vi "wr_xively_one_element.vi"(1 "VALUE":dbl, 2 "Xively_name":string) -> ()   [LabVIEW 2012]
uses:
  <vilib>/httpClient/LabVIEWHTTPClient.lvlib
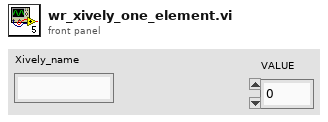
[diagram p1: front panel]
types:
  T1 = typedef "LabVIEWHTTPClient.lvlib/ClientHandle.ctl" = refnum<k1>
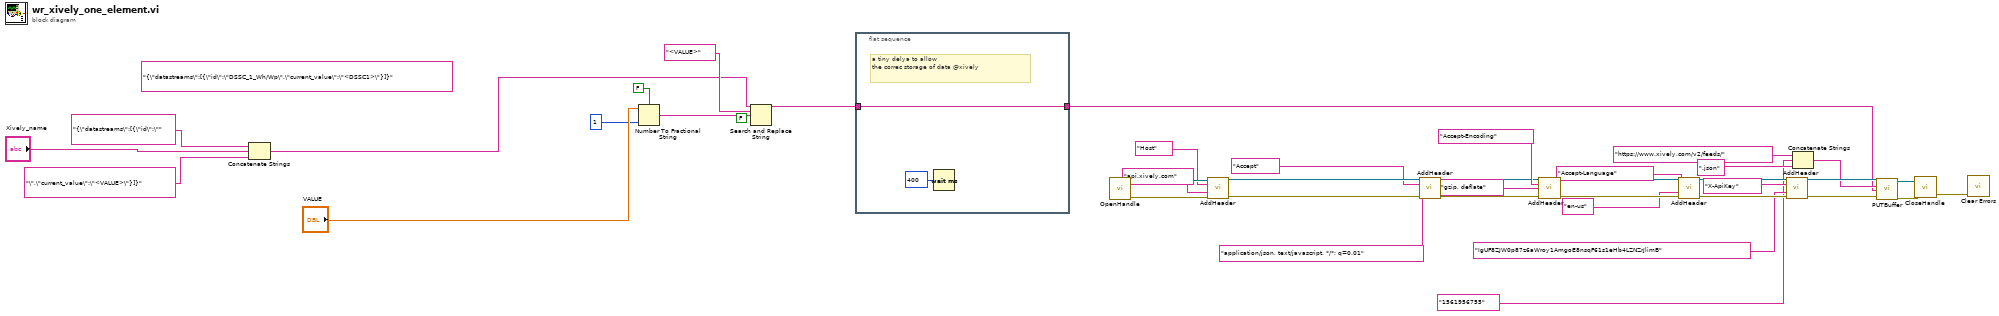
[diagram p0: block diagram]
diagram:
  (unwired) FALSE ("use system decimal point (T)")
  (unwired) "{\"datastreams\":[{\"id\":\"DSSC_1_Wh/Wp\",\"current_value\":\"<DSSC1>\"}]}" ("input string")
  n1 = Concatenate Strings("{\"datastreams\":[{\"id\":\"" ("input string"), "Xively_name", "\",\"current_value\":\"<VALUE>\"}]}" ("input string")) -> (w3:string)
  n2 = Number To Fractional String(use system decimal point (T)=FALSE, number="VALUE", precision (6)=i16 1) -> (F-format string=w18:string)  [unwired: 1 in]
  n3 = Search and Replace String(input string=w3, search string="<VALUE>", replace string=w18) -> (result string=w2:string)  [unwired: 5 in, 3 out]
  n4 = flat-sequence {
    tunnel: w2 -> [w42]
    tunnel: [w42] -> w1
    frame #0 {
      # "a tiny delya to allow\nthe correc storage of data @xively"
      n5 = Wait (ms)(milliseconds to wait=u32 400) -> ()  [unwired: 1 out]
    }
  }
  n6 = call <vilib>:"OpenHandle.vi"() -> ("client handle out"=w36:T1, "error out"=w35:errorcluster)  [unwired: 14 in]
  n7 = call <vilib>:"AddHeader.vi"("client handle"=w36, "header"="Host", "value"="api.xively.com", "error in (no error)"=w35) -> ("client handle out"=w32:T1, "error out"=w31:errorcluster)  [unwired: 10 in]
  n8 = call <vilib>:"AddHeader.vi"("client handle"=w32, "header"="Accept", "value"="application/json, text/javascript, */*; q=0.01", "error in (no error)"=w31) -> ("client handle out"=w27:T1, "error out"=w26:errorcluster)  [unwired: 10 in]
  n9 = call <vilib>:"AddHeader.vi"("client handle"=w27, "header"="Accept-Encoding", "value"="gzip, deflate", "error in (no error)"=w26) -> ("client handle out"=w24:T1, "error out"=w23:errorcluster)  [unwired: 10 in]
  n10 = call <vilib>:"AddHeader.vi"("client handle"=w24, "header"="Accept-Language", "value"="en-us", "error in (no error)"=w23) -> ("client handle out"=w20:T1, "error out"=w19:errorcluster)  [unwired: 10 in]
  n11 = call <vilib>:"AddHeader.vi"("client handle"=w20, "header"="X-ApiKey", "value"="IgUF8ZJW0p87z6aWroy1AmgoE8nsqF61s1eHb4LZNZrJlimB" ("API Key"), "error in (no error)"=w19) -> ("client handle out"=w39:T1, "error out"=w38:errorcluster)  [unwired: 10 in]
  n12 = Concatenate Strings("https://www.xively.com/v2/feeds/" ("url"), "1561956755" ("Feed ID"), ".json" ("string")) -> (w15:string)
  n13 = call <vilib>:"PUTBuffer.vi"("client handle"=w39, "url"=w15, "buffer"=w1, "error in (no error)"=w38) -> ("client handle out"=w14:T1, "error out"=w13:errorcluster)  [unwired: 8 in, 2 out]
  n14 = call <vilib>:"CloseHandle.vi"("client handle"=w14, "error in (no error)"=w13) -> ("error out"=w9:errorcluster)  [unwired: 13 in]
  n15 = call <vilib>:"Clear Errors.vi"("error in (no error)"=w9) -> ()  [unwired: 6 in, 1 out]
